vi "IIR Cascade Filter with I.C..vi"   [LabVIEW 2020, in "NI_AALBase.lvlib"]
doc: "Filters the input sequence <B>X</B> using the cascade form of the IIR filter specified by the <B>IIR Filter Cluster</B>. This VI is similar to the IIR Cascade Filter VI except that you specify the initial conditions for this VI. Wire data to the <B>X</B> input to determine the polymorphic instance to use or manually select the instance."
uses:
  NI_AALBase.lvlib
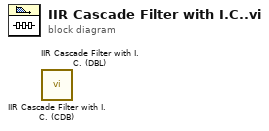
[diagram p0: block diagram]
diagram:
  n1 = call "IIR Cascade Filter with I.C. (CDB).vi"() -> ()  [unwired: 3 in, 3 out]
  n2 = call "IIR Cascade Filter with I.C. (DBL).vi"() -> ()  [unwired: 3 in, 3 out]
